vi "RFSwitch.vi"(4 "Controller Device Description":string="DLP-IO20", 5 "RF Channel":u32=4 min=1 max=4 step=1) -> (2 "OK":bool)   [LabVIEW 2018]
uses:
  Rf switch/Write-Read Byte Array Demo 7.0/Global 1.vi
panel:
  out "Ping result":u8 format="%x"
  out "Status":i32=1
  out "Bytes Written 6":i32=5
  out "Bytes Read 6":i32
  out "Read Array 6":i32[](array[numeric])
  out "Write Array 6":i32[](array[numeric])=[5, 53, 6, 0, 0]
  out "Bytes Written 7":i32=5
  out "Bytes Read 7":i32
  out "Read Array 7":i32[](array[numeric])
  out "Write Array 7":i32[](array[numeric])=[5, 53, 7, 0, 0]
  out "Handle":u64=263961288
  # "RF switch control panel"
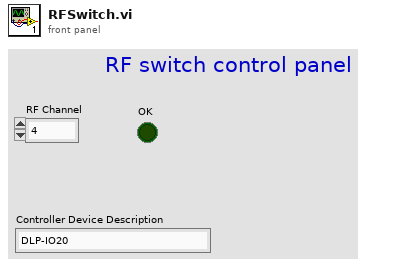
[diagram p1: front panel]
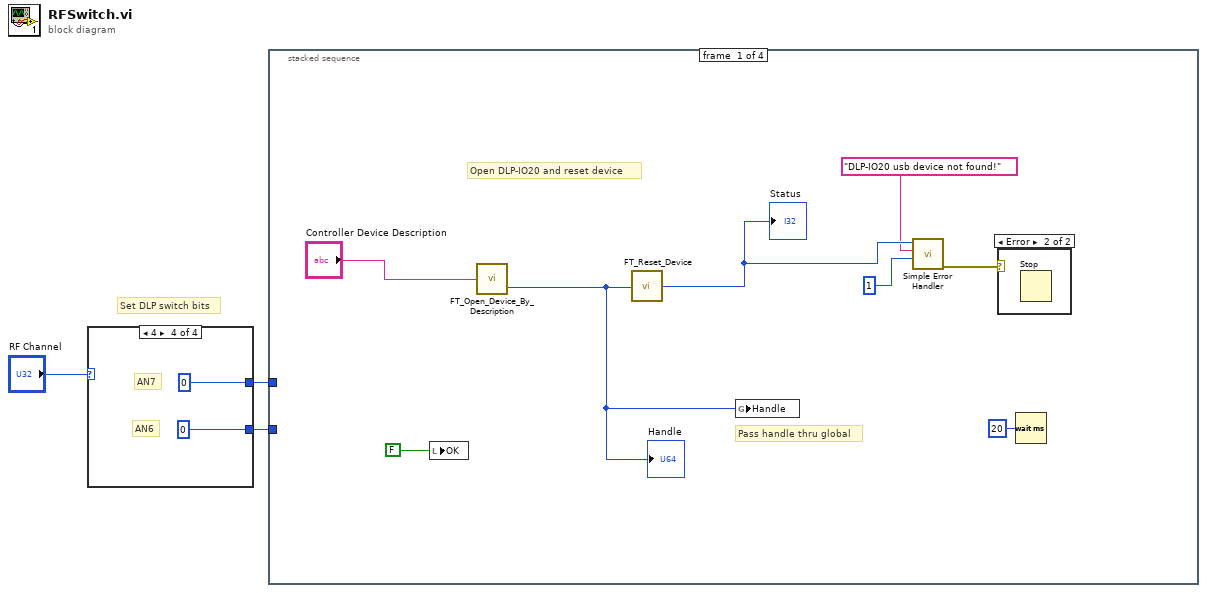
[diagram p0: block diagram]
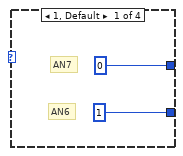
[diagram p2: hidden frame]
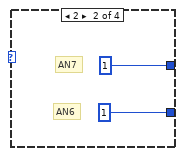
[diagram p3: hidden frame]
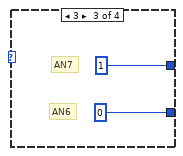
[diagram p4: hidden frame]
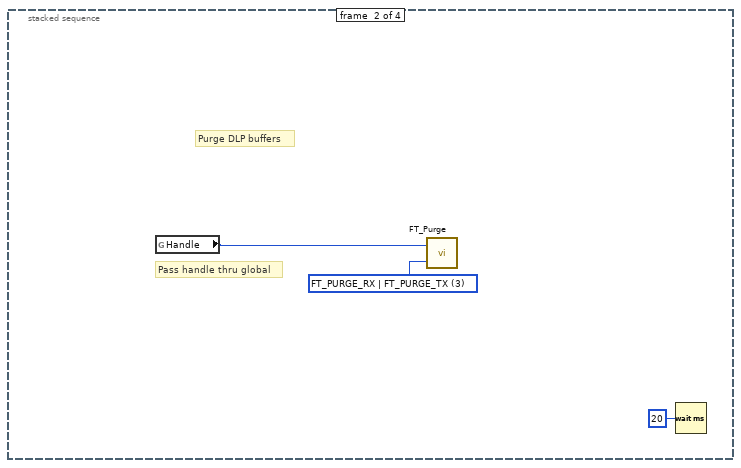
[diagram p6: hidden frame]
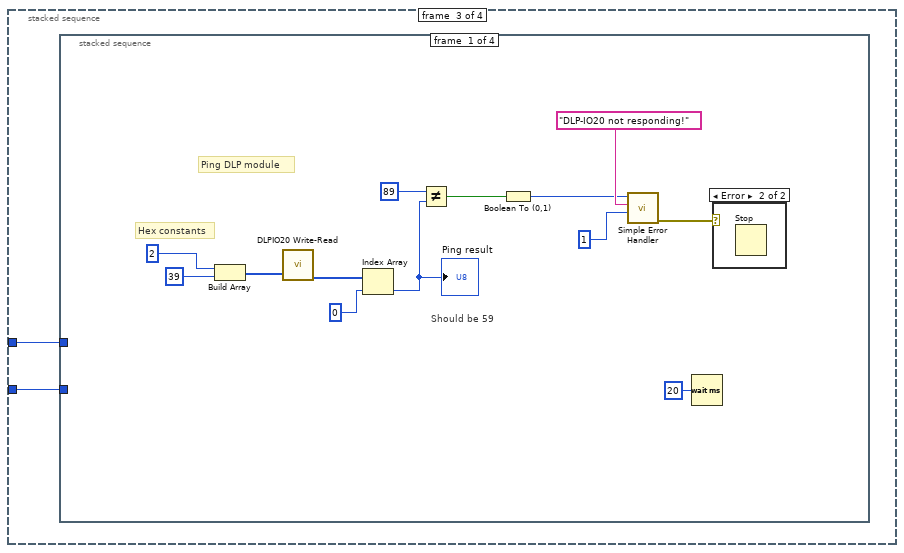
[diagram p7: hidden frame]
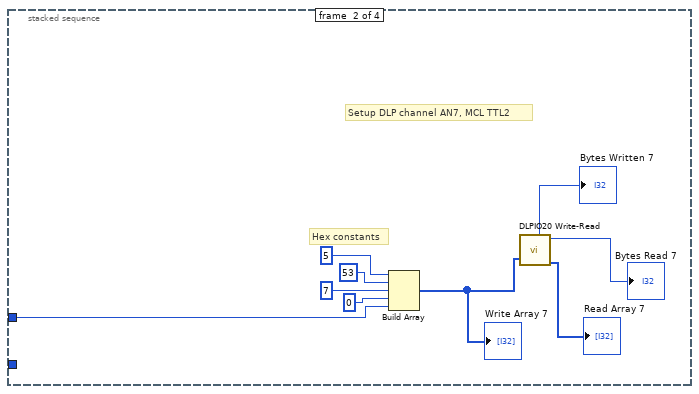
[diagram p9: hidden frame]
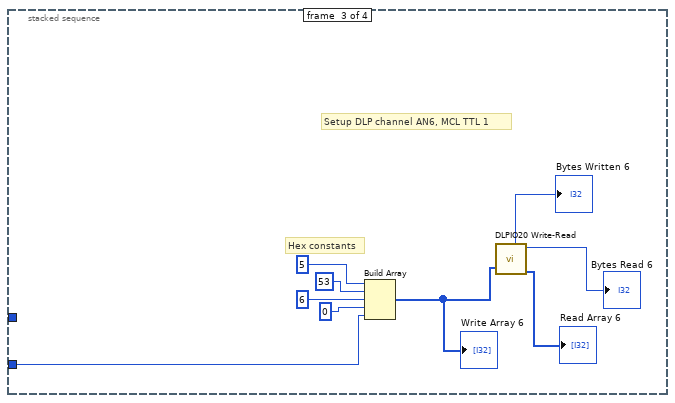
[diagram p10: hidden frame]
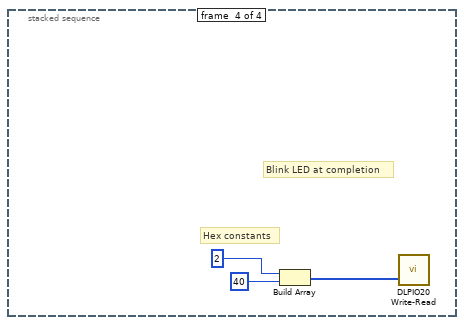
[diagram p11: hidden frame]
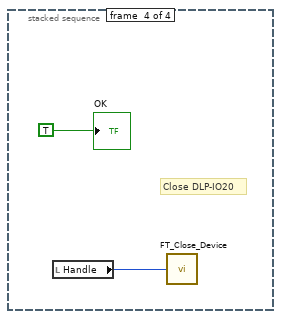
[diagram p12: hidden frame]
diagram:
  # "Set DLP switch bits"
  n1 = case shown="4" "RF Channel" {
    tunnel: [0 1 1 0] -> w2
    tunnel: [1 1 0 0] -> w1
    frame 1, Default {
      # "AN6"
      # "AN7"
    }
    frame 2 {
      # "AN6"
      # "AN7"
    }
    frame 3 {
      # "AN6"
      # "AN7"
    }
    frame 4 {
      # "AN6"
      # "AN7"
    }
  }
  n2 = stacked-sequence {
    tunnel: w2 -> [_ _ w24 _]
    tunnel: w1 -> [_ _ w23 _]
    frame #0 {
      # "Pass handle thru global"
      # "Open DLP-IO20 and reset device"
      n3 = local write "OK"(FALSE) -> ()
      n4 = call "FT_Open_Device_By_Description.vi"("Device Description"="Controller Device Description") -> ("Handle"=w17:u64)  [unwired: 1 out]
      "Handle" <- w17
      n5 = call "FT_Reset_Device.vi"("Handle"=w17) -> ("FT_Status"=w16:u32)
      "Status" <- w16
      n6 = global write "Global 1.vi" "Handle"(w17) -> ()
      n7 = call <vilib>:"Simple Error Handler.vi"("error code (no error:0)"=w16, "error source (\" \")"="DLP-IO20 usb device not found!", "type of dialog (OK msg:1)"=1) -> ("error out"=w13:errorcluster)  [unwired: 2 in, 4 out]
      n8 = case shown="Error" w13 {
        frame No Error {
        }
        frame Error {
          n9 = Stop() -> ()  [unwired: 1 in]
        }
      }
      n10 = Wait (ms)(milliseconds to wait=u32 20) -> ()  [unwired: 1 out]
    }
    frame #1 {
      w22 = u32 3 items=["FT_PURGE_RX"=1, "FT_PURGE_TX"=2, "FT_PURGE_RX | FT_PURGE_TX"=3] ("Purge Flags")
      # "Purge DLP buffers"
      # "Pass handle thru global"
      n11 = global read "Global 1.vi" "Handle"() -> (w21:u64)
      n12 = call "FT_Purge.vi"("Purge Flags"=w22, "Handle"=w21) -> ()  [unwired: 1 out]
      n13 = Wait (ms)(milliseconds to wait=u32 20) -> ()  [unwired: 1 out]
    }
    frame #2 {
      n14 = stacked-sequence {
        tunnel: w24 -> [_ w38 _ _]
        tunnel: w23 -> [_ _ w47 _]
        frame #0 {
          # "Should be 59"
          # "Ping DLP module"
          # "Hex constants"
          n15 = Build Array "Build Array"(u8 2, u8 39) -> (w35:u8[])
          n16 = call "DLPIO20 Write-Read.vi"("Write Buffer"=w35) -> ("Read Buffer Out"=w34:u8[])  [unwired: 3 in, 2 out]
          n17 = Index Array(array=w34, index=u8 0) -> (element=w31:u8)
          "Ping result" <- w31
          n18 = Not Equal?(x=u8 89, y=w31) -> (x != y?=w27:bool)
          n19 = Boolean To (0,1)(Boolean=w27) -> (0, 1=w26:i16)
          n20 = call <vilib>:"Simple Error Handler.vi"("error code (no error:0)"=w26, "error source (\" \")"="DLP-IO20 not responding!", "type of dialog (OK msg:1)"=1) -> ("error out"=w28:errorcluster)  [unwired: 2 in, 4 out]
          n21 = Wait (ms)(milliseconds to wait=u32 20) -> ()  [unwired: 1 out]
          n22 = case shown="Error" w28 {
            frame No Error {
            }
            frame Error {
              n23 = Stop() -> ()  [unwired: 1 in]
            }
          }
        }
        frame #1 {
          # "Setup DLP channel AN7, MCL TTL2"
          # "Hex constants"
          n24 = Build Array "Build Array"(u8 5, u8 53, u8 7, u8 0, w38) -> (w41:i32[])
          "Write Array 7" <- w41
          n25 = call "DLPIO20 Write-Read.vi"("Write Buffer"=w41) -> ("Read Buffer Out"=→"Read Array 7":u8[], "Bytes Read"=→"Bytes Read 7":u32, "Bytes Written"=→"Bytes Written 7":u32)  [unwired: 3 in]
        }
        frame #2 {
          # "Setup DLP channel AN6, MCL TTL 1"
          # "Hex constants"
          n26 = Build Array "Build Array"(u8 5, u8 53, u8 6, u8 0, w47) -> (w50:i32[])
          "Write Array 6" <- w50
          n27 = call "DLPIO20 Write-Read.vi"("Write Buffer"=w50) -> ("Read Buffer Out"=→"Read Array 6":u8[], "Bytes Read"=→"Bytes Read 6":u32, "Bytes Written"=→"Bytes Written 6":u32)  [unwired: 3 in]
        }
        frame #3 {
          # "Blink LED at completion"
          # "Hex constants"
          n28 = Build Array "Build Array"(u8 2, u8 40) -> (w56:u8[])
          n29 = call "DLPIO20 Write-Read.vi"("Write Buffer"=w56) -> ()  [unwired: 3 in, 3 out]
        }
      }
    }
    frame #3 {
      # "Close DLP-IO20"
      n30 = local read "Handle"() -> (w60:u64)
      n31 = call "FT_Close_Device.vi"("Handle"=w60) -> ()  [unwired: 1 out]
      "OK" <- TRUE
    }
  }
